vi "UT_EField_DAQ_AnalogIO.emergency off.vi"(0 "i ref in":refnum<vi>, 3 "Timeout":i32=10000, 5 "error in":errorcluster caption="Fehler (Eingang, kein Fehler)") -> (14 "i ref out":refnum<vi>, 17 "timed out":bool, 19 "error out":errorcluster caption="Fehler (Ausgang)")   [LabVIEW 2014, in "UT_EField_DAQ_AnalogIO.lvlib"]
doc: "Contact: Falk Ziegler, eMail: info@lab-coding.de"
uses:
  UT_EField_DAQ_AnalogIO.lvlib
  CS_Core/CSApplicationBaseClasses/DeviceBase/DeviceBase.lvlib
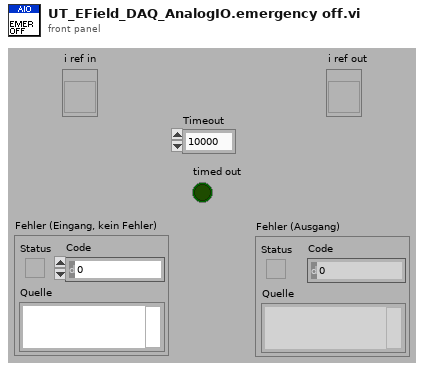
[diagram p1: front panel]
types:
  T1 = typedef "UT_EField_DAQ_AnalogIO.lvlib/UT_EField_DAQ_AnalogIO.i attribute.ctl" = cluster{"inputs":cluster{"index":i32[], "channel_task":refnum<k21>[], "range":cluster{"min":dbl, "max":dbl}[], "channel_number":i32, "scale_factor":dbl}, "outputs":cluster{"index":i32[], "channel_task":refnum<k21>[], "range":cluster{"min":dbl, "max":dbl}[], "channel_number":i32, "scale_factor":dbl}}
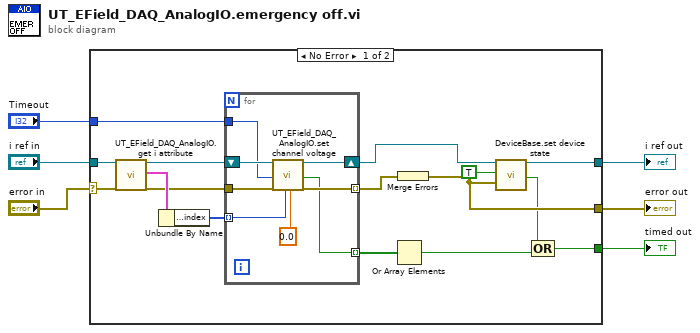
[diagram p0: block diagram]
diagram:
  n1 = case shown="No Error" "error in" {
    selector: "error in" -> [w20 w31]
    tunnel: "i ref in" -> [w19 w32]
    tunnel: [w22 w32] -> w4
    tunnel: "Timeout" -> [w15 _]
    tunnel: [w12 w31] -> w2
    tunnel: [w7 _] -> w1
    frame No Error {
      n2 = call "UT_EField_DAQ_AnalogIO.get i attribute.vi"("i ref in"=w19, "error in (no error)"=w20) -> ("i ref out"=w16:refnum<vi>, "i attribute"=w18:T1, "error out"=w13:errorcluster)  [unwired: 15 in]
      n3 = Unbundle By Name(w18) -> ("outputs.index"=w17:i32[])
      n4 = for {
        tunnel: w17 -> [w23] mode=indexing
        tunnel: [w29] -> w14 mode=indexing
        tunnel: w15 -> [w28]
        tunnel: w13 -> [w27]
        shift-right: [w26] -> w11
        shift-left: w16 -> [w30]
        tunnel: [w25] -> w10 mode=indexing
        n5 = call "UT_EField_DAQ_AnalogIO.set channel voltage.vi"("i ref in"=w30, "Timeout"=w28, "error in"=w27, "channel_index"=w23, "voltage"=0.0) -> ("i ref out"=w26:refnum<vi>, "timed out"=w25:bool, "error out"=w29:errorcluster)  [unwired: 12 in]
      }
      n6 = Or Array Elements(Boolean array=w10) -> (logical OR=w8:bool)
      n7 = Merge Errors(w14) -> (w12:errorcluster)
      n8 = call "DeviceBase.set device state.vi"("i ref in"=w11, "implicit"=TRUE, "device error"=w12) -> ("i ref out"=w22:refnum<vi>, "timed out"=w9:bool)  [unwired: 14 in, 1 out]
      n9 = Compound Arithmetic op=OR(w9, w8) -> (w7:bool)
    }
    frame Error {
    }
  }
  "error out" <- w2
  "timed out" <- w1
  "i ref out" <- w4
